vi "Set VI To Display.vi"(8 "error in (no error)":errorcluster, 10 "Display Size":cluster{"Width":i16, "Height":i16}, 11 "VI In":refnum<vi>) -> (0 "error out":errorcluster, 2 "Found":bool, 3 "VI":refnum<vi>)   [LabVIEW 2022 SP3, in "TouchControl.lvlib"]
uses:
  TouchControl.lvlib
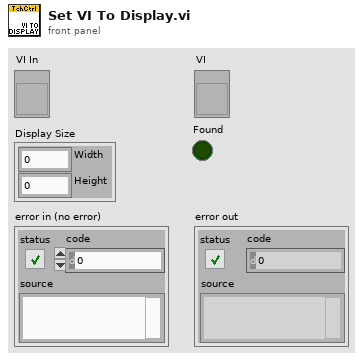
[diagram p1: front panel]
types:
  T1 = typedef "LVAllMonitorsDisplayTypeDef.ctl" = cluster{"Bounds":cluster{"Left":i16, "Top":i16, "Right":i16, "Bottom":i16}, "Depth":i16}[]
  T2 = cluster{"Left":i16, "Top":i16, "Right":i16, "Bottom":i16}
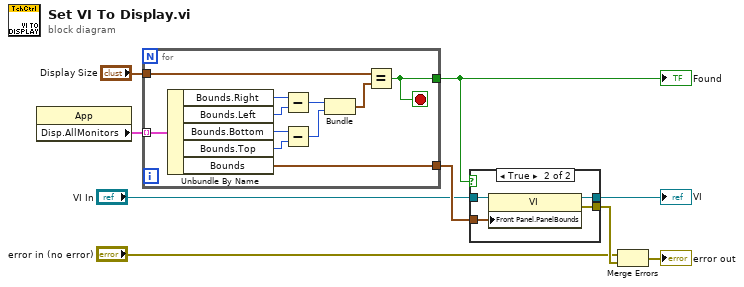
[diagram p0: block diagram]
diagram:
  n1 = property class="App"() -> ("Disp.AllMonitors"=w9:T1)  [unwired: 2 in, 2 out]
  n2 = for {
    tunnel: w9 -> [w20] mode=indexing
    tunnel: [w19] -> w7
    tunnel: "Display Size" -> [w12]
    tunnel: [w10] -> w6
    stop <- w10 stop-if-true
    n3 = Unbundle By Name(w20) -> ("Bounds.Right"=w18:i16, "Bounds.Left"=w17:i16, "Bounds.Bottom"=w16:i16, "Bounds.Top"=w15:i16, "Bounds"=w19:T2)
    n4 = Subtract(x=w18, y=w17) -> (x-y=w14:i16)
    n5 = Subtract(x=w16, y=w15) -> (x-y=w13:i16)
    n6 = Bundle(w14, w13) -> (w11:cluster{i16, i16})  [unwired: 1 in]
    n7 = Equal?(x=w12, y=w11) -> (x = y?=w10:bool)
  }
  "Found" <- w6
  n8 = case shown="True" w6 {
    tunnel: "VI In" -> [w21 w25]
    tunnel: w7 -> [_ w24]
    tunnel: [_ w23] -> w4
    tunnel: [w21 w22] -> w1
    frame False {
    }
    frame True {
      n9 = property class="VI"(reference=w25, "Front Panel.PanelBounds"=w24) -> (reference out=w22:refnum<vi>, error out=w23:errorcluster)  [unwired: 1 in]
    }
  }
  "VI" <- w1
  n10 = Merge Errors("error in (no error)", w4) -> (→"error out":errorcluster)
